vi "LabVIEW Code_SCADA_Speed Control_DC Motor.vi"() -> ()   [LabVIEW 2018]
uses:
  <vilib>/addons/Control Design/_Model Construction/Data Typedefs.llb/CD Variables.ctl
  <vilib>/Instr/_visa.llb/VISA Configure Serial Port (Instr).vi
  <vilib>/addons/control/pid/pid.llb/PID (DBL).vi
  <vilib>/addons/Control Design/_Model Construction/Model Creation.llb/Model Creation SubVI/cd_Create Symbolic Transfer Function Model.vi
  <vilib>/addons/Control Design/_Time Response Analysis/Time Response.llb/Time Response subVI/cd_Step Response (Transfer Function).vi
  <vilib>/addons/Control Design/_Frequency Response Analysis/Frequency Response.llb/Frequency Response subVI/cd_Bode (Transfer Function).vi
  <vilib>/addons/Control Design/_Utility/Model Viewer.llb/Model Viewer SubVI/cd_Draw Transfer Function Equation (TF).vi
  <vilib>/addons/control/pid/NI_PID_pid.lvlib
  <vilib>/addons/Control Design/_Model Construction/NI_LinSys_Model Creation.lvlib
  <vilib>/addons/Control Design/_Utility/NI_CD_Model Viewer.lvlib
  <vilib>/addons/Control Design/_Frequency Response Analysis/NI_CD_Frequency Response.lvlib
  <vilib>/addons/Control Design/_Time Response Analysis/NI_CD_Time Response.lvlib
  <vilib>/addons/Control Design/_Model Construction/NI_LinSys_Data Typedefs.lvlib
panel:
  in  "Tab Control":enum32{"Page 1", "Page 2"}(tab)
  in  "?":bool
  in  "?":refnum<visa-resource-name>
  out "vitesse reelle":dbl(knob) scale=0.0..160.0
  in  "Consigne":i32(slide) scale=0.0..160.0
  in  "PID gains":T1={"K (Proportionnel)"=1.0, "Ki (Integrateur)"=0.01, "Kd (Dérivateur)"=0.0} {"Kd (Dérivateur)" scale=0.0..10.0; "Ki (Integrateur)" scale=0.0..10.0; "K (Proportionnel)" scale=0.0..10.0}
  out "Consigne/Vitesse réelle(tr/min)":dynamicdata(graph)
  in  "Variales du numérateur":string[](array[string])
  in  "Variables du dénominateur":string[](array[string])
  in  "Variables":T2 {"Value" format="%.2f"}
  out "Equation":picture
  out "Diagramme de bode de gain":cluster{"W":dbl[], "Magnitude":dbl[]}[](graph)
  out "Diagramme de bode de phase":cluster{"W":dbl[], "Magnitude":dbl[]}[](graph)
  out "Reponse inditielle":cluster{"time":dbl[], dbl[]}[](graph)
  # "Systeme SCADA pour le controle de vitesse d'un moteur DC"
  # "Fonction de transfert est du premier ordre:\n        Numerateur: K                      avec       K=0,028 .\n        Dénominateur:  K^2 + J*Rm  avec J=9,64E-6  et Rm=3,3"
  # "Etude de la fonction de transfert du moteur"
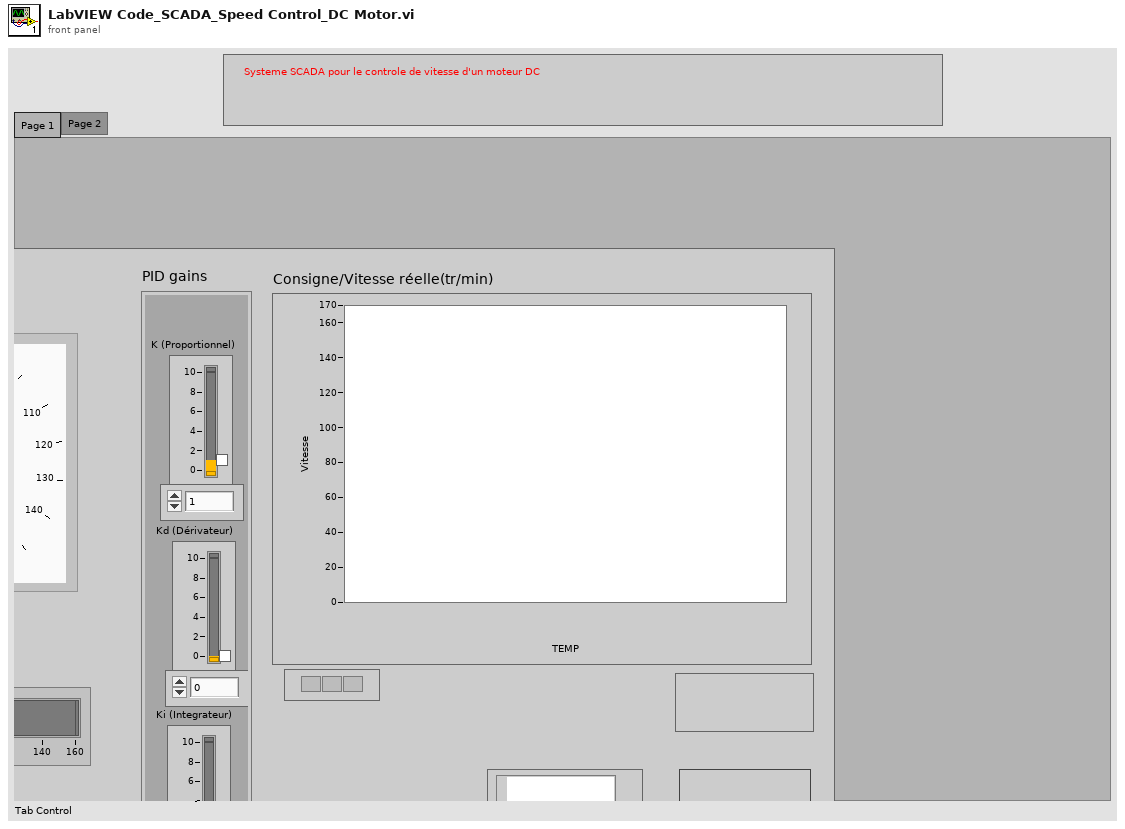
[diagram p1: front panel]
types:
  T1 = cluster{"K (Proportionnel)":dbl, "Ki (Integrateur)":dbl, "Kd (Dérivateur)":dbl}
  T2 = typedef "NI_LinSys_Data Typedefs.lvlib/CD Variables.ctl" = cluster{"Name":string, " Value":dbl}[]
  T3 = typedef "NI_LinSys_Model Typedefs.lvlib/CD Transfer Function Model (MIMO).ctl" = cluster{"properties":T4, "transfer function(s)":T5[][]}
  T4 = typedef "NI_LinSys_Model Typedefs.lvlib/CD General Elements.ctl" = cluster{"Model name":string, "Input names":string[], "Output names":string[], "Input Delays":dbl[], "Output Delays":dbl[], "Sampling Time":dbl, "Notes":string}
  T5 = typedef "NI_LinSys_Model Typedefs.lvlib/CD Transfer Function Model (SISO).ctl" = cluster{"Numerator":dbl[], "Denominator":dbl[], "delay":dbl}
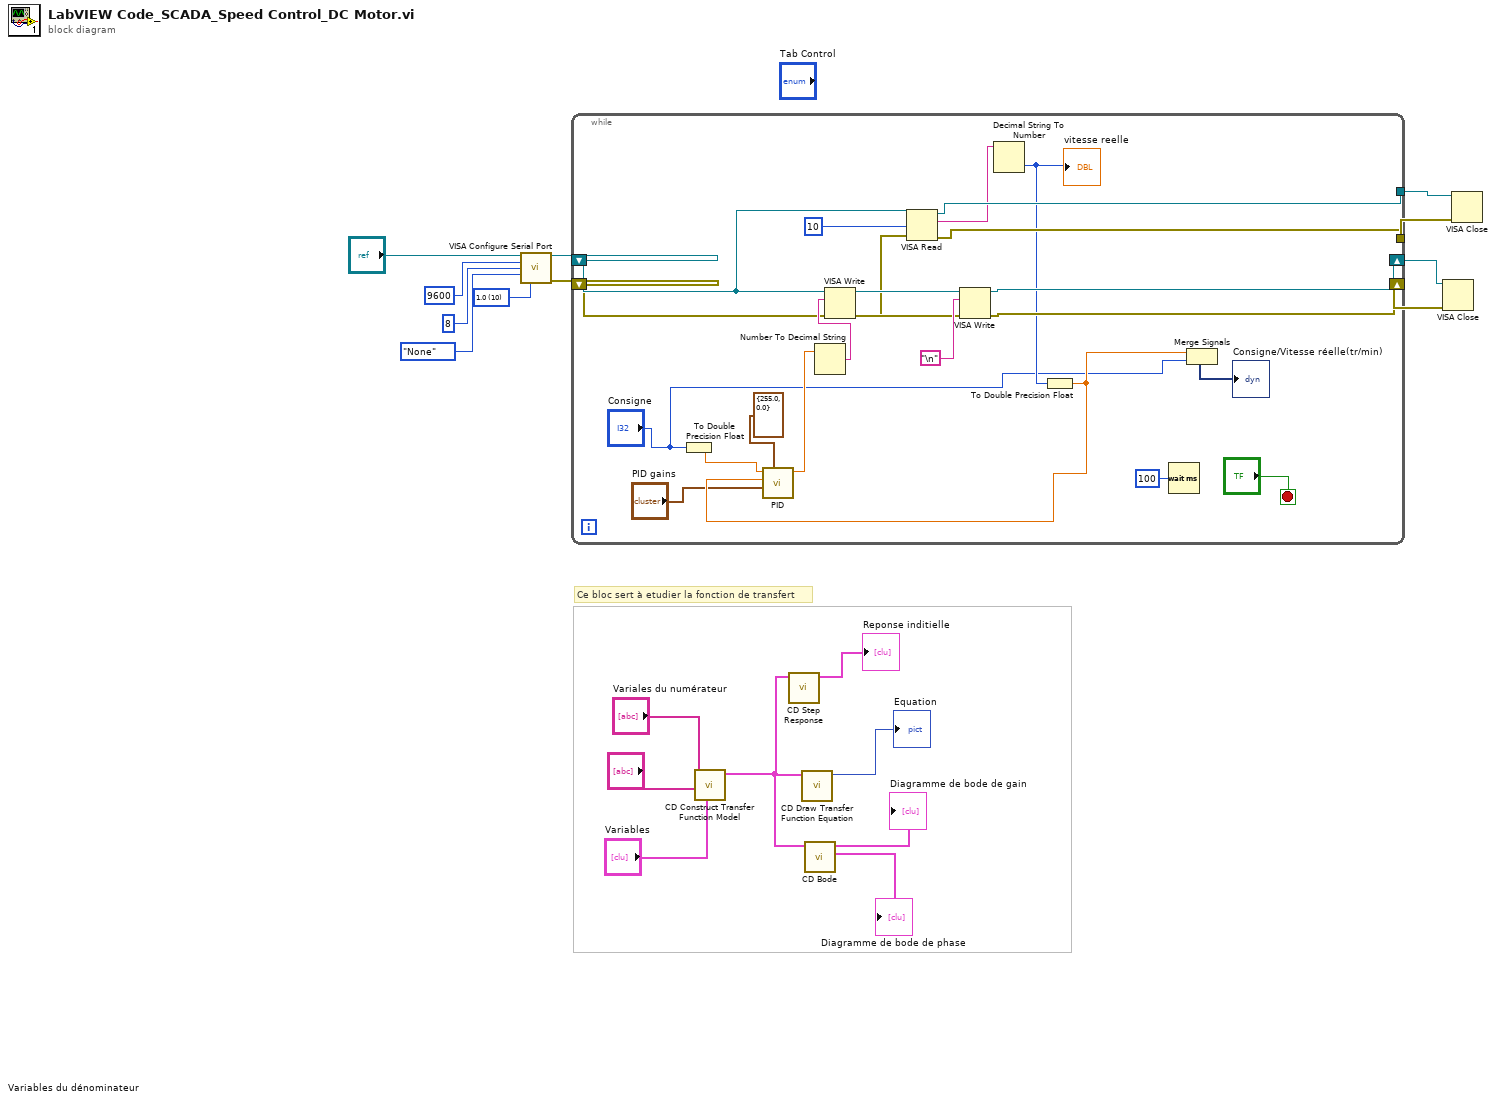
[diagram p0: block diagram]
diagram:
  w14 = u16 10 items=["1.0"=10, "1.5"=15, "2.0"=20] ("stop bits (10: 1 bit)")
  # "Ce bloc sert à etudier la fonction de transfert"
  n1 = call-poly "VISA Configure Serial Port"("VISA resource name"="?", "baud rate (9600)"=u32 9600, "data bits (8)"=u16 8, "parity (0:none)"=enum16{"None", "Odd", "Even", "Mark", "Space"}."None", "stop bits (10: 1 bit)"=w14) -> ("VISA resource name out"=w13:refnum<visa-resource-name>, "error out"=w12:errorcluster)  [unwired: 9 in]
  n2 = while {
    shift-right: [w35] -> w2
    shift-left: w13 -> [w33]
    shift-right: [w34] -> w19
    shift-left: w12 -> [w32]
    tunnel: [w31] -> w11
    tunnel: [w30] -> w1
    stop <- "?" stop-if-true
    n3 = To Double Precision Float(number="Consigne") -> (double precision float=w27:dbl)
    n4 = VISA Read(VISA resource name=w33, byte count=u32 10, error in (no error)=w32) -> (VISA resource name out=w31:refnum<visa-resource-name>, read buffer=w28:string, error out=w30:errorcluster)  [unwired: 1 out]
    n5 = Decimal String To Number(string=w28) -> (number=w26:i32)  [unwired: 2 in, 1 out]
    "vitesse reelle" <- w26
    n6 = To Double Precision Float(number=w26) -> (double precision float=w23:dbl)
    n7 = call-poly <vilib>:"PID.vi"("output range"=cluster{"output high":dbl, "output low":dbl} {"output high"=255.0, "output low"=0.0}, "PID gains"="PID gains", "process variable"=w23, "setpoint"=w27) -> ("output"=w24:dbl)  [unwired: 6 in, 1 out]
    n8 = Number To Decimal String(number=w24) -> (decimal integer string=w36:string)  [unwired: 1 in]
    n9 = VISA Write(VISA resource name=w33, write buffer=w36, error in (no error)=w32) -> (VISA resource name out=w38:refnum<visa-resource-name>, error out=w37:errorcluster)  [unwired: 1 out]
    n10 = VISA Write(VISA resource name=w38, write buffer="\n", error in (no error)=w37) -> (VISA resource name out=w35:refnum<visa-resource-name>, error out=w34:errorcluster)  [unwired: 1 out]
    n11 = Wait (ms)(milliseconds to wait=u32 100) -> ()  [unwired: 1 out]
    n12 = Merge Signals(w23, "Consigne") -> (→"Consigne/Vitesse réelle(tr/min)":dynamicdata)
  }
  n13 = call-poly <vilib>:"CD Construct Transfer Function Model.vi"("Variables"="Variables", "Symbolic Denominator"="Variables du dénominateur", "Symbolic Numerator"="Variales du numérateur") -> ("Transfer Function Model"=w4:T3)  [unwired: 7 in, 1 out]
  n14 = call-poly <vilib>:"CD Step Response.vi"("Transfer Function Model"=w4) -> ("Step Response Graph"=→"Reponse inditielle":cluster{"time":dbl[], dbl[]}[])  [unwired: 8 in, 2 out]
  n15 = call-poly <vilib>:"CD Draw Transfer Function Equation.vi"("Transfer Function Model"=w4) -> ("Equation"=→"Equation":picture)  [unwired: 8 in, 2 out]
  n16 = call-poly <vilib>:"CD Bode.vi"("Transfer Function Model"=w4) -> ("Bode Phase"=→"Diagramme de bode de phase":cluster{"W":dbl[], "Magnitude":dbl[]}[], "Bode Magnitude"=→"Diagramme de bode de gain":cluster{"W":dbl[], "Magnitude":dbl[]}[])  [unwired: 6 in, 3 out]
  n17 = VISA Close(VISA resource name=w2, error in (no error)=w19) -> ()  [unwired: 1 out]
  n18 = VISA Close(VISA resource name=w11, error in (no error)=w1) -> ()  [unwired: 1 out]
